vi "Sub Init UI.vi"(8 "error in (no error)":errorcluster, 11 "LF2R IDE in":refnum<class "LF2R IDE.lvclass">) -> (0 "error out":errorcluster, 3 "LF2R IDE out":refnum<class "LF2R IDE.lvclass">)   [LabVIEW 2018, in "LF2R IDE.lvlib" / "LF2R IDE.lvclass"]
uses:
  LF2R IDE.lvclass
  LF2R IDE.lvclass/LF2R IDE.ctl
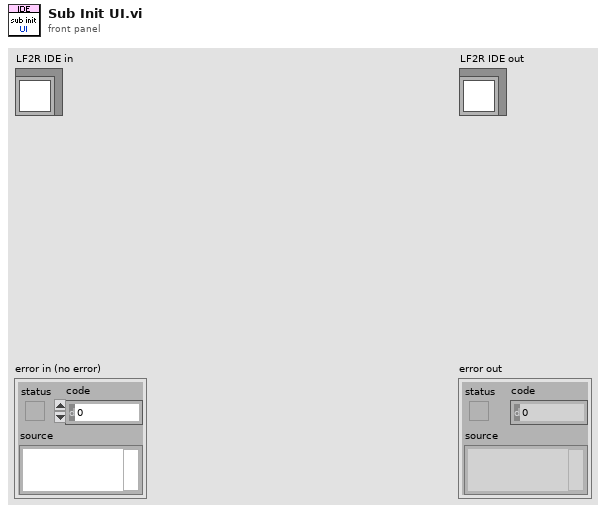
[diagram p1: front panel]
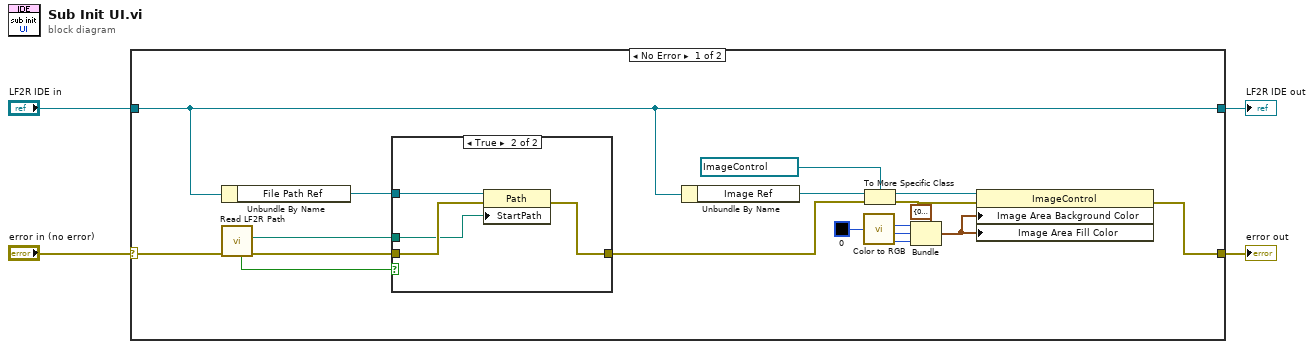
[diagram p0: block diagram]
diagram:
  n1 = case shown="No Error" "error in (no error)" {
    selector: "error in (no error)" -> [w20 w29]
    tunnel: [w5 w29] -> w3
    tunnel: [w17 w28] -> w1
    tunnel: "LF2R IDE in" -> [w17 w28]
    frame No Error {
      n2 = Unbundle By Name(w17) -> ("File Path Ref"=w22:refnum<vi>)
      n3 = call "Read LF2R Path.vi"("error in (no error)"=w20) -> ("error out"=w21:errorcluster, "Data Path"=w19:path, "Found"=w18:bool)  [unwired: 6 in, 2 out]
      n4 = case shown="True" w18 {
        tunnel: w22 -> [_ w27]
        tunnel: w21 -> [w23 w26]
        tunnel: w19 -> [_ w25]
        tunnel: [w23 w24] -> w6
        frame False {
        }
        frame True {
          n5 = property class="Path"(reference=w27, error in=w26, "StartPath"=w25) -> (error out=w24:errorcluster)  [unwired: 1 out]
        }
      }
      n6 = Unbundle By Name(w17) -> ("Image Ref"=w10:refnum<vi>)
      n7 = call <vilib>:"Color to RGB.vi"("Color"=u32 0) -> ("R"=w15:u8, "G"=w14:u8, "B"=w13:u8)  [unwired: 1 out]
      n8 = To More Specific Class(target class=refnum<vi> refnum ("reference"), reference=w10, error in=w6) -> (specific class reference=w9:refnum<vi>, error out=w7:errorcluster)
      n9 = Bundle(cluster=cluster{"Red":u8, "Green":u8, "Blue":u8} {"Red"=0, "Green"=0, "Blue"=0} ("Image Area:Background:Background Color"), "Red"=w15, "Green"=w14, "Blue"=w13) -> (w11:cluster{"Red":u8, "Green":u8, "Blue":u8})
      n10 = property class="ImageControl"(reference=w9, error in=w7, "Image Area Background Color"=w11, "Image Area Fill Color"=w11) -> (error out=w5:errorcluster)  [unwired: 1 out]
    }
    frame Error {
    }
  }
  "error out" <- w3
  "LF2R IDE out" <- w1
